vi "AWG Stop Pulses.vi"(8 "error in (no error)":errorcluster, 11 "awg session in":T1) -> (0 "error out":errorcluster, 3 "awg session out":T1)   [LabVIEW 2018, in "AWG.lvlib"]
doc: "AWG wrapper: Stops generation of pulses at output. At least for 33120 model this should be called first after initialization to stop standard waveform mode, i.e. to stop output."
uses:
  AWG.lvlib
  AWG Session.ctl
  AWG Type.ctl
  Agilent 33XXX Series/Agilent 33XXX Series.lvlib
  AFG3000/Tektronix AFG 3000 Series.lvlib
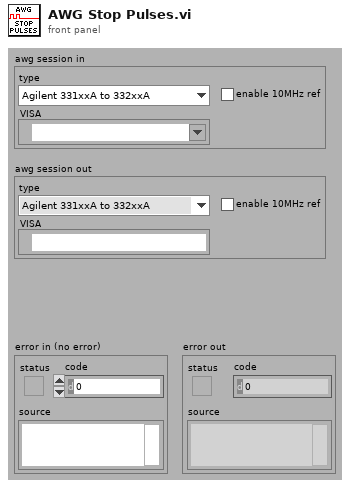
[diagram p1: front panel]
types:
  T1 = typedef "AWG.lvlib/AWG Session.ctl" = cluster{"type":T2, "VISA":refnum<visa-resource-name>, "enable 10MHz ref":bool}
  T2 = typedef "AWG.lvlib/AWG Type.ctl" = enum16{"Agilent 331xxA to 332xxA", "Agilent 335xxA to 336xxA", "Tektronix AFG3101C", "dummy"}
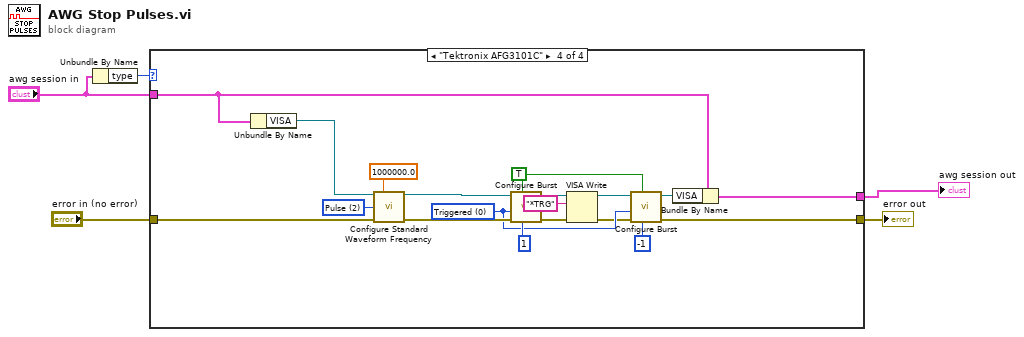
[diagram p0: block diagram]
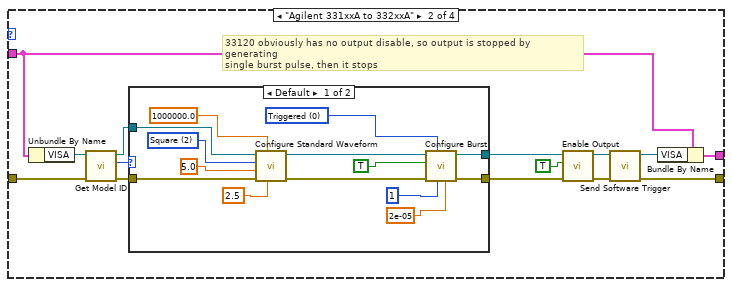
[diagram p3: hidden frame]
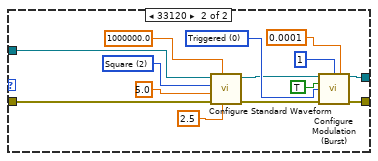
[diagram p4: hidden frame]
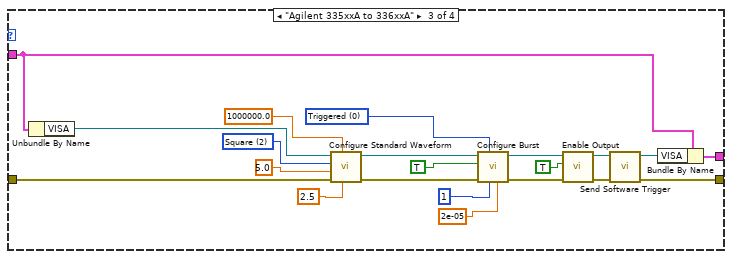
[diagram p5: hidden frame]
diagram:
  n1 = Unbundle By Name("awg session in") -> ("type"=w5:T2)
  n2 = case shown="\"Tektronix AFG3101C\"" w5 {
    tunnel: "error in (no error)" -> [w7 w19 w50 w86]
    tunnel: [w7 w8 w62 w76] -> w3
    tunnel: "awg session in" -> [w6 w20 w70 w88]
    tunnel: [w6 w21 w69 w87] -> w1
    frame Default {
    }
    frame "Agilent 331xxA to 332xxA" {
      # "33120 obviously has no output disable, so output is stopped by generating\nsingle burst pulse, then it stops"
      n3 = Unbundle By Name(w20) -> ("VISA"=w18:refnum<visa-resource-name>)
      n4 = call "Get Model ID.vi"("error in (no error)"=w19, "VISA resource name"=w18) -> ("error out"=w17:errorcluster, "model ID"=w15:u32, "VISA resource name out"=w16:refnum<visa-resource-name>)  [unwired: 7 in]
      n5 = case shown="Default" w15 {
        tunnel: [w31 w45] -> w13
        tunnel: [w30 w44] -> w12
        tunnel: w17 -> [w25 w43]
        tunnel: w16 -> [w24 w42]
        frame Default {
          w27 = u16 2 items=["DC", "Sine", "Square", "Triangle", "Ramp", "Pulse", "Noise", "Sinc", "Negative Ramp", "Exponential Rise", "Exponential Fall", "Cardiac"] ("Waveform Function (1: Sine)")
          w35 = u16 0 items=["Triggered", "Gated"] ("Burst Mode (0: Triggered)")
          n6 = call "Configure Standard Waveform.vi"("DC Offset (0.00 V)"=2.5, "Frequency (1000 Hz)"=1000000.0, "error in (no error)"=w25, "Amplitude (1)"=5.0, "Waveform Function (1: Sine)"=w27, "VISA resource name"=w24) -> ("error out"=w23:errorcluster, "VISA resource name out"=w22:refnum<visa-resource-name>)  [unwired: 4 in]
          n7 = call "Configure Burst.vi"("Burst Period (1 s)"=2e-05, "Burst Count (1)"=1, "Burst Mode (0: Triggered)"=w35, "error in (no error)"=w23, "Enable Burst (T: Enable)"=TRUE, "VISA resource name"=w22) -> ("error out"=w31:errorcluster, "VISA resource name out"=w30:refnum<visa-resource-name>)  [unwired: 4 in]
        }
        frame 33120 {
          w38 = u16 2 items=["DC", "Sine", "Square", "Triangle", "Ramp", "Pulse", "Noise", "Sinc", "Negative Ramp", "Exponential Rise", "Exponential Fall", "Cardiac"] ("Waveform Function (1: Sine)")
          w46 = u16 0 items=["Triggered", "Gated"] ("Burst Modulation Mode (0: Triggered)")
          n8 = call "Configure Standard Waveform.vi"("DC Offset (0.00 V)"=2.5, "Frequency (1000 Hz)"=1000000.0, "error in (no error)"=w43, "Amplitude (1)"=5.0, "Waveform Function (1: Sine)"=w38, "VISA resource name"=w42) -> ("error out"=w41:errorcluster, "VISA resource name out"=w40:refnum<visa-resource-name>)  [unwired: 4 in]
          n9 = call "Configure Modulation (Burst).vi"("VISA resource name"=w40, "Burst Count (1)"=1, "Burst Period (1 s)"=0.0001, "Enable Burst Modulation (T: Enable)"=TRUE, "Burst Modulation Mode (0: Triggered)"=w46, "error in (no error)"=w41) -> ("VISA resource name out"=w44:refnum<visa-resource-name>, "error out"=w45:errorcluster)  [unwired: 8 in]
        }
      }
      n10 = call "Enable Output.vi"("error in (no error)"=w13, "Enable Output  (T: Enable)"=TRUE, "VISA resource name"=w12) -> ("error out"=w11:errorcluster, "VISA resource name out"=w10:refnum<visa-resource-name>)  [unwired: 7 in]
      n11 = call "Send Software Trigger.vi"("error in (no error)"=w11, "VISA resource name"=w10) -> ("error out"=w8:errorcluster, "VISA resource name out"=w9:refnum<visa-resource-name>)  [unwired: 8 in]
      n12 = Bundle By Name(cluster=w20, "VISA"=w9) -> (w21:T1)
    }
    frame "Agilent 335xxA to 336xxA" {
      w55 = u16 2 items=["DC", "Sine", "Square", "Triangle", "Ramp", "Pulse", "Noise", "Sinc", "Negative Ramp", "Exponential Rise", "Exponential Fall", "Cardiac"] ("Waveform Function (1: Sine)")
      w61 = u16 0 items=["Triggered", "Gated"] ("Burst Mode (0: Triggered)")
      n13 = Unbundle By Name(w70) -> ("VISA"=w51:refnum<visa-resource-name>)
      n14 = call "Configure Standard Waveform.vi"("DC Offset (0.00 V)"=2.5, "Frequency (1000 Hz)"=1000000.0, "error in (no error)"=w50, "Amplitude (1)"=5.0, "Waveform Function (1: Sine)"=w55, "VISA resource name"=w51) -> ("error out"=w53:errorcluster, "VISA resource name out"=w52:refnum<visa-resource-name>)  [unwired: 4 in]
      n15 = call "Configure Burst.vi"("Burst Period (1 s)"=2e-05, "Burst Count (1)"=1, "Burst Mode (0: Triggered)"=w61, "error in (no error)"=w53, "Enable Burst (T: Enable)"=TRUE, "VISA resource name"=w52) -> ("error out"=w67:errorcluster, "VISA resource name out"=w66:refnum<visa-resource-name>)  [unwired: 4 in]
      n16 = call "Enable Output.vi"("error in (no error)"=w67, "Enable Output  (T: Enable)"=TRUE, "VISA resource name"=w66) -> ("error out"=w65:errorcluster, "VISA resource name out"=w64:refnum<visa-resource-name>)  [unwired: 7 in]
      n17 = call "Send Software Trigger.vi"("error in (no error)"=w65, "VISA resource name"=w64) -> ("error out"=w62:errorcluster, "VISA resource name out"=w63:refnum<visa-resource-name>)  [unwired: 8 in]
      n18 = Bundle By Name(cluster=w70, "VISA"=w63) -> (w69:T1)
    }
    frame "Tektronix AFG3101C" {
      w81 = u16 2 items=["Sine", "Square", "Pulse", "Ramp", "Noise", "DC", "Sin(x)/x", "Gaussian", "Lorentz", "Exponential Rise", "Exponential Decay", "Haversine"] ("Waveform Function (0: Sine)")
      w79 = TRUE ("Enable Burst (T: Enable)")
      w78 = u16 0 items=["Triggered", "Gated"] ("Burst Mode (0: Triggered)")
      n19 = Unbundle By Name(w88) -> ("VISA"=w83:refnum<visa-resource-name>)
      n20 = call "Configure Standard Waveform Frequency.vi"("VISA resource name"=w83, "Frequency (1000 Hz)"=1000000.0, "Waveform Function (0: Sine)"=w81, "error in (no error)"=w86) -> ("VISA resource name out"=w84:refnum<visa-resource-name>, "error out"=w85:errorcluster)  [unwired: 10 in]
      n21 = call "Configure Burst.vi"("Burst Count (5)"=1, "Enable Burst (T: Enable)"=w79, "error in (no error)"=w85, "Burst Mode (0: Triggered)"=w78, "VISA resource name"=w84) -> ("error out"=w75:errorcluster, "VISA resource name out"=w74:refnum<visa-resource-name>)  [unwired: 5 in]
      n22 = VISA Write(VISA resource name=w74, write buffer="*TRG", error in (no error)=w75) -> (VISA resource name out=w73:refnum<visa-resource-name>, error out=w72:errorcluster)  [unwired: 1 out]
      n23 = call "Configure Burst.vi"("Burst Count (5)"=-1, "Enable Burst (T: Enable)"=w79, "error in (no error)"=w72, "Burst Mode (0: Triggered)"=w78, "VISA resource name"=w73) -> ("error out"=w76:errorcluster, "VISA resource name out"=w77:refnum<visa-resource-name>)  [unwired: 5 in]
      n24 = Bundle By Name(cluster=w88, "VISA"=w77) -> (w87:T1)
    }
  }
  "error out" <- w3
  "awg session out" <- w1
